vi "HMP_ReadCurrent.vi"(8 "error in (no error)":errorcluster, 10 "Channel (Channel 1)":i32(ring)=1 items=["Channel 1"=1, "Channel 2"=2, "Channel 3"=3, "Channel 4"=4], 11 "HMP VISA In":refnum<visa-resource-name> caption="VISA resource name") -> (0 "error out":errorcluster, 3 "Current Value":dbl format="%.3f")   [LabVIEW 2022 SP3]
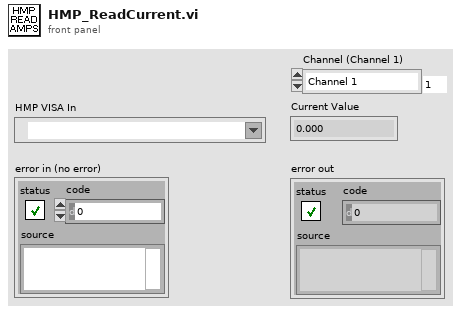
[diagram p1: front panel]
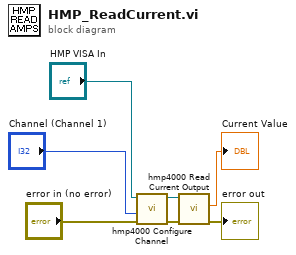
[diagram p0: block diagram]
diagram:
  n1 = call "hmp4000 Configure Channel.vi"("error in (no error)"="error in (no error)", "Channel (Channel 1)"="Channel (Channel 1)", "VISA resource name"="HMP VISA In") -> ("error out"=w1:errorcluster, "VISA resource name out"=w2:refnum<visa-resource-name>)  [unwired: 7 in]
  n2 = call "hmp4000 Read Current Output.vi"("error in (no error)"=w1, "VISA resource name"=w2) -> ("error out"=→"error out":errorcluster, "Current Value"=→"Current Value":dbl)  [unwired: 7 in, 1 out]
